vi "Create Message Queue.vi"(0 "message queue name":string, 1 "max queue size (-1, unlimited)":i32=-1, 5 "initial message names":string[](array[string]), 7 "initial message values":string[](array[string]), 11 "error in":errorcluster) -> (4 "message queue out":T1, 15 "error out":errorcluster)   [LabVIEW 2014, in "AMC.lvlib"]
doc: "Creates a new local message queue or returns a reference to an existing message queue baseed on the queue name. You can pass in a list of initial messages which will be added to the queue."
uses:
  AMC.lvlib
  Message Queue.ctl
  Message.ctl
  <vilib>/NI/Tools/Keyed Array/KeyedArray.ctl
  <vilib>/NI/Tools/Keyed Array/Tools_KeyedArray.lvlib
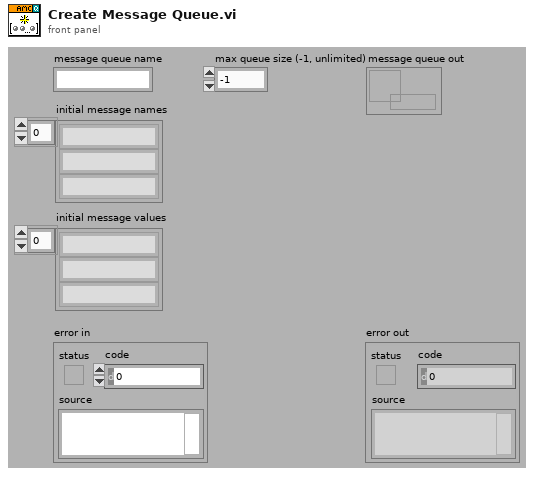
[diagram p1: front panel]
types:
  T1 = typedef "AMC.lvlib/Message Queue.ctl" = refnum<queue>
  T2 = typedef "AMC.lvlib/Message.ctl" = cluster{"name":string, "value":string, "attributes":T3, "receiver host":string, "receiver process":string, "source host":string, "source process":string, "priority message":bool, "acknowledge message":bool}
  T3 = typedef "Tools_KeyedArray.lvlib/KeyedArray.ctl" = cluster{"keys":string[], "values":string[]}
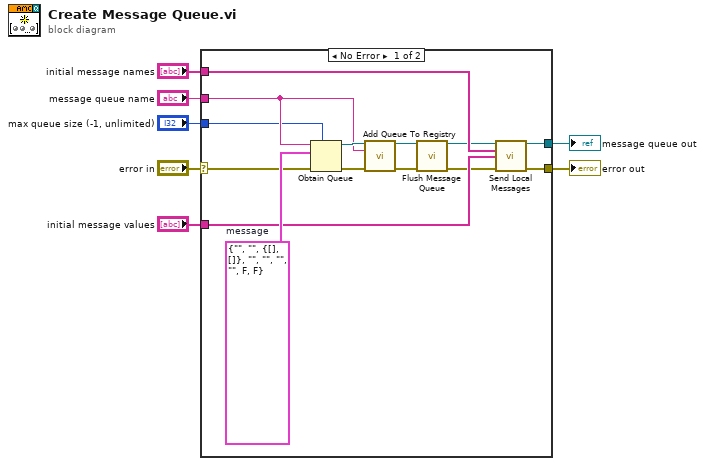
[diagram p0: block diagram]
diagram:
  n1 = case shown="No Error" "error in" {
    selector: "error in" -> [w8 w22]
    tunnel: [w20 w22] -> w7
    tunnel: [w19 _] -> w6
    tunnel: "initial message names" -> [w18 _]
    tunnel: "initial message values" -> [w17 _]
    tunnel: "message queue name" -> [w14 _]
    tunnel: "max queue size (-1, unlimited)" -> [w9 _]
    frame No Error {
      w21 = T2 {"name"="", "value"="", "attributes"={"keys"=[], "values"=[]}, "receiver host"="", "receiver process"="", "source host"="", "source process"="", "priority message"=FALSE, "acknowledge message"=FALSE}  # message
      n2 = Obtain Queue(max queue size (-1, unlimited)=w9, name (unnamed)=w14, element data type=w21, error in (no error)=w8) -> (queue out=w15:refnum<queue>, error out=w16:errorcluster)  [unwired: 1 in, 1 out]
      n3 = call "Add Queue To Registry.vi"("message queue in"=w15, "name"=w14, "error in"=w16) -> ("message queue out"=w12:T1, "error out"=w13:errorcluster)  [unwired: 11 in]
      n4 = call "Flush Message Queue.vi"("message queue in"=w12, "error in"=w13) -> ("message queue out"=w11:T1, "error out"=w10:errorcluster)  [unwired: 11 in, 1 out]
      n5 = call "Send Local Messages.vi"("message queue in"=w11, "message names"=w18, "message values"=w17, "error in"=w10) -> ("message queue out"=w19:T1, "error out"=w20:errorcluster)  [unwired: 9 in, 1 out]
    }
    frame Error {
    }
  }
  "message queue out" <- w6
  "error out" <- w7
